vi "总磷总氮测量数据储存.vi"   [LabVIEW 2016, in "斯坦道通用流路CODmn.lvlib"]
uses:
  <vilib>/ptbypt/NI_PtbyPt.lvlib
types:
  T1 = cluster{"跨度值":dbl, "零点标准液浓度":dbl, "跨度标准液浓度":dbl, "标准液标准浓度":dbl}
  T2 = cluster{"系统时间":timestamp, "工作状态":u16, "测量模式":enum16{"待机", "连续模式", "周期模式", "定点模式", "受控模式", "手动模式"}, "告警代码":u16, "故障代码":u16, "日志代码":u16, "软件版本":u16, "F0":sgl, "F1":sgl, "F2":sgl, "F3":sgl, "T":sgl, "H":sgl, "id":u16, "flowid":u16, "量程":u16, "总磷控温温度1":sgl, "营养盐控温温度2":sgl, "ADC":sgl}
  T3 = cluster{"运行模式":enum16{"维护模式", "常规模式", "应急模式", "质控模式"}, "质控频次":enum16{"关闭", "每天", "星期一", "星期二", "星期三", "星期四", "星期五", "星期六", "星期日"}, "空白核查时间":u16, "跨度核查时间":u16, "测量间隔":u16}
  T4 = cluster{"总磷跨度值":dbl, "总磷零点标准液浓度":dbl, "总磷跨度标准液浓度":dbl, "总磷标准液标准浓度":dbl, "总氮跨度值":dbl, "总氮零点标准液浓度":dbl, "总氮跨度标准液浓度":dbl, "总氮标准液标准浓度":dbl, "COD跨度值":dbl, "COD零点标准液浓度":dbl, "COD跨度标准液浓度":dbl, "COD标准液标准浓度":dbl, "氨氮跨度值":dbl, "氨氮零点标准液浓度":dbl, "氨氮跨度标准液浓度":dbl, "氨氮标准液标准浓度":dbl, "磷酸盐跨度值":dbl, "磷酸盐零点标准液浓度":dbl, "磷酸盐跨度标准液浓度":dbl, "磷酸盐标准液标准浓度":dbl, "硝氮跨度值":dbl, "硝氮零点标准液浓度":dbl, "硝氮跨度标准液浓度":dbl, "硝氮标准液标准浓度":dbl, "亚硝氮跨度值":dbl, "亚硝氮零点标准液浓度":dbl, "亚硝氮跨度标准液浓度":dbl, "亚硝氮标准液标准浓度":dbl, "硫化物跨度值":dbl, "硫化物零点标准液浓度":dbl, "硫化物跨度标准液浓度":dbl, "硫化物标准液标准浓度":dbl, "硅酸盐跨度值":dbl, "硅酸盐零点标准液浓度":dbl, "硅酸盐跨度标准液浓度":dbl, "硅酸盐标准液标准浓度":dbl, "总磷零点标准液偏差":dbl, "总磷跨度标准液偏差":dbl, "总磷标准液标准偏差":dbl, "总氮零点标准液偏差":dbl, "总氮跨度标准液偏差":dbl, "总氮标准液标准偏差":dbl, "COD零点标准液偏差":dbl, "COD跨度标准液偏差":dbl, "COD标准液标准偏差":dbl, "氨氮零点标准液偏差":dbl, "氨氮跨度标准液偏差":dbl, "氨氮标准液标准偏差":dbl, "磷酸盐零点标准液偏差":dbl, "磷酸盐跨度标准液偏差":dbl, "磷酸盐标准液标准偏差":dbl, "硝氮零点标准液偏差":dbl, "硝氮跨度标准液偏差":dbl, "硝氮标准液标准偏差":dbl, "亚硝氮零点标准液偏差":dbl, "亚硝氮跨度标准液偏差":dbl, "亚硝氮标准液标准偏差":dbl, "硫化物零点标准液偏差":dbl, "硫化物跨度标准液偏差":dbl, "硫化物标准液标准偏差":dbl, "硅酸盐零点标准液偏差":dbl, "硅酸盐跨度标准液偏差":dbl, "硅酸盐标准液标准偏差":dbl, "氟化物跨度值":dbl, "氟化物零点标准液浓度":dbl, "氟化物跨度标准液浓度":dbl, "氟化物标准液标准浓度":dbl, "氟化物零点标准液偏差":dbl, "氟化物跨度标准液偏差":dbl, "氟化物标准液标准偏差":dbl, "CODMn跨度值":dbl, "CODMn零点标准液浓度":dbl, "CODMn跨度标准液浓度":dbl, "CODMn标准液标准浓度":dbl, "CODMn零点标准液偏差":dbl, "CODMn跨度标准液偏差":dbl, "CODMn标准液标准偏差":dbl}
  T5 = cluster{"因子编码":u32, "单位":u16, "标样参考值":sgl, "水样数据时间":timestamp, "水样实测值":sgl, "水样数据标识":string, "标样数据时间":timestamp, "标样实测值":sgl, "标样数据标识":string, "空白数据时间":timestamp, "空白实测值":sgl, "空白数据标识":string, "零点核查数据时间":timestamp, "零点核查实测值":sgl, "零点核查数据标识":string, "跨度核查数据时间":timestamp, "跨度核查实测值":sgl, "跨度核查数据标识":string, "加标回收数据时间":timestamp, "加标回收实测值":sgl, "加标回收数据标识":string, "平行样数据时间":timestamp, "平行样实测值":sgl, "平行样数据标识":string, "F0":sgl, "F1":sgl, "F2":sgl, "F3":sgl, "F4":sgl, "F5":sgl, "F6":sgl, "F7":sgl, "温度":sgl, "湿度":sgl, "X值":sgl, "fidrange":u16, "X1值":sgl}[]
  T6 = enum16{"水样测试", "标样核查", "跨度核查", "零点核查", "加标回收", "空白测试", "平行样"}[]
  T7 = cluster{"因子编码":u32, "单位":u16, "标样参考值":sgl, "水样数据时间":timestamp, "水样实测值":sgl, "水样数据标识":string, "标样数据时间":timestamp, "标样实测值":sgl, "标样数据标识":string, "空白数据时间":timestamp, "空白实测值":sgl, "空白数据标识":string, "零点核查数据时间":timestamp, "零点核查实测值":sgl, "零点核查数据标识":string, "跨度核查数据时间":timestamp, "跨度核查实测值":sgl, "跨度核查数据标识":string, "加标回收数据时间":timestamp, "加标回收实测值":sgl, "加标回收数据标识":string, "平行样数据时间":timestamp, "平行样实测值":sgl, "平行样数据标识":string, "F0":sgl, "F1":sgl, "F2":sgl, "F3":sgl, "F4":sgl, "F5":sgl, "F6":sgl, "F7":sgl, "温度":sgl, "湿度":sgl, "X值":sgl, "fidrange":u16, "X1值":sgl}
  T8 = cluster{"时间标识":timestamp, "测量模式":enum16{"维护数据", "水样测试", "标样核查", "零点核查", "跨度核查", "空白测试", "平行样测试", "加标回收", "空白校准", "标样校准", "初始化（清洗）", "快捷测试"}, "数据标记表":string, "监测值":sgl, "单位":u16, "数据标识":string, "因子编码":u32, "标样参考值":sgl, "F0":sgl, "F1":sgl, "F2":sgl, "F3":sgl, "F4":sgl, "F5":sgl, "F6":sgl, "F7":sgl, "X":sgl, "温度":sgl, "湿度":sgl, "量程标识":string, "SN":string, "跨度值":sgl, "X1":sgl}
  T9 = typedef "斯坦道通用流路CODmn.lvlib/关键参数.ctl" = cluster{"测量量程":sgl, "测量检出限":sgl, "测量精度":sgl, "测量间隔":sgl, "消解温度":sgl, "消解时长":sgl, "三项式系数":sgl, "二次多项式系数":sgl, "曲线斜率":sgl, "曲线截距":sgl, "线性相关系数":sgl, "空白校准时间":timestamp, "标样校准时间":timestamp, "测量信号值":sgl, "稀释倍数":sgl, "空白标定系数":sgl, "量程系数":sgl}
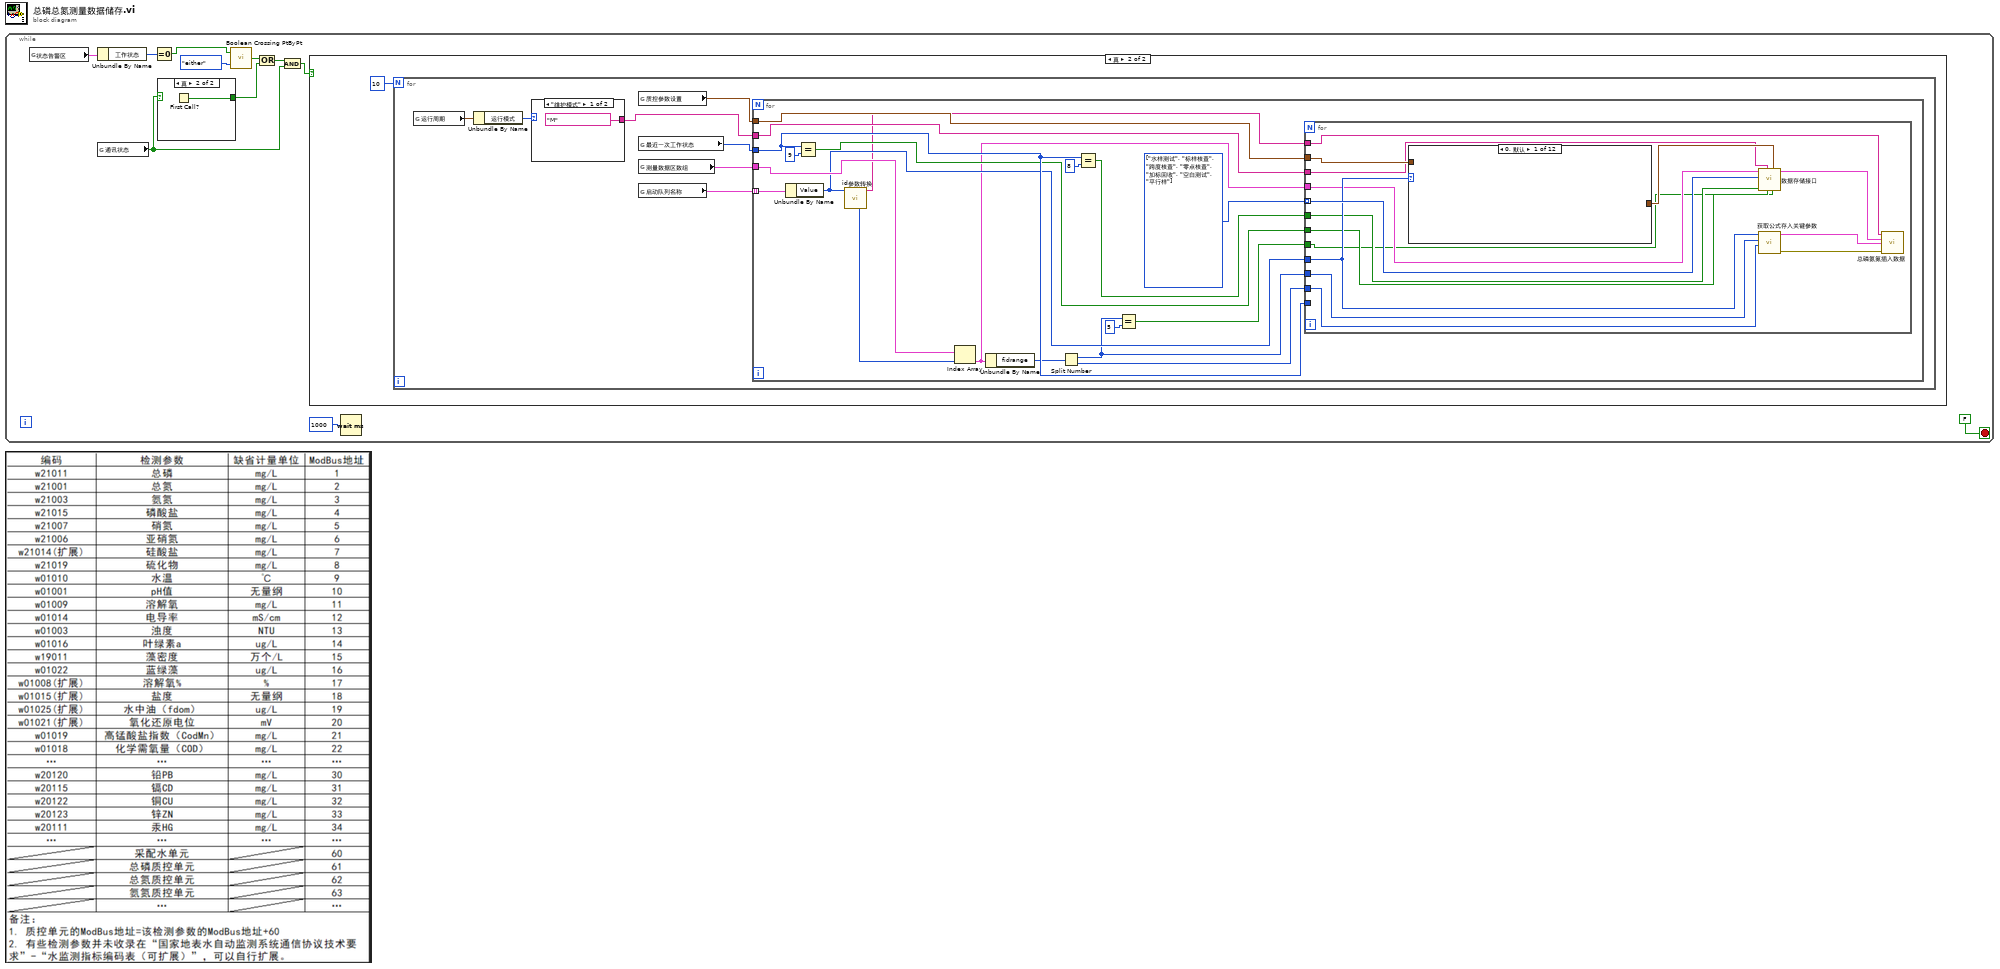
[diagram p0: block diagram]
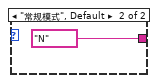
[diagram p4: hidden frame]
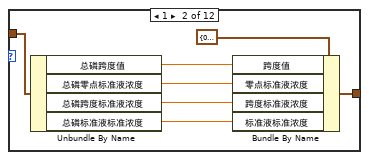
[diagram p5: hidden frame]
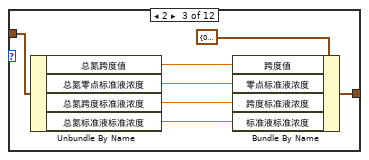
[diagram p6: hidden frame]
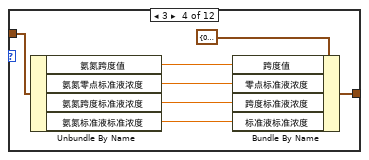
[diagram p7: hidden frame]
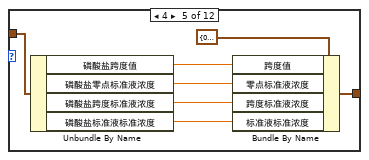
[diagram p8: hidden frame]
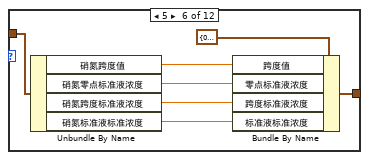
[diagram p9: hidden frame]
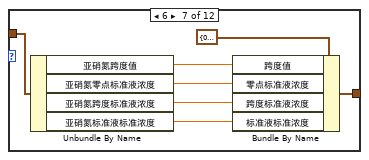
[diagram p10: hidden frame]
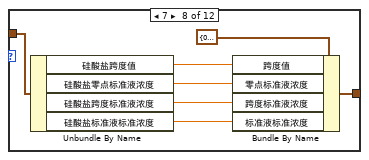
[diagram p11: hidden frame]
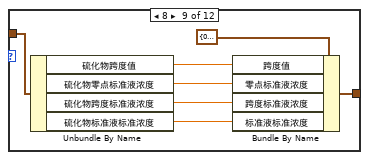
[diagram p12: hidden frame]
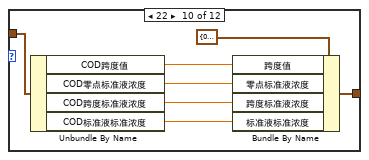
[diagram p13: hidden frame]
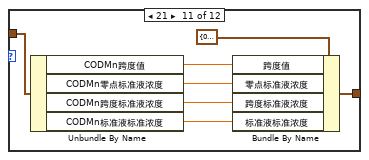
[diagram p14: hidden frame]
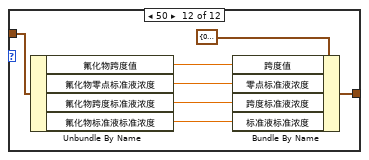
[diagram p15: hidden frame]
diagram:
  n1 = while {
    stop <- FALSE stop-if-true
    n2 = global read "VAR总磷总氮全局变量.vi" "状态告警区"() -> (w10:T2)
    n3 = Unbundle By Name(w10) -> ("工作状态"=w8:u16)
    n4 = global read "VAR总磷总氮全局变量.vi" "通讯状态"() -> (w3:bool)
    n5 = Equal To 0?(x=w8) -> (x = 0?=w5:bool)
    n6 = case shown="真" w3 {
      tunnel: [_ w12] -> w1
      frame False {
      }
      frame True {
        n7 = First Call?() -> (First Call?: T/F=w12:bool)
      }
    }
    n8 = call <vilib>:"Boolean Crossing PtByPt.vi"("direction"=enum16{"either", "false-true", "true-false"}."either", "input"=w5) -> ("crossing"=w6:bool)  [unwired: 1 in]
    n9 = Or(x=w6, y=w1) -> (x .or. y?=w2:bool)
    n10 = And(x=w2, y=w3) -> (x .and. y?=w4:bool)
    n11 = case shown="真" w4 {
      frame False {
      }
      frame True {
        n12 = for {
          N: 10 -> [_]
          n13 = global read "总磷总氮断电保存全局变量.vi" "运行周期"() -> (w16:T3)
          n14 = Unbundle By Name(w16) -> ("运行模式"=w15:enum16{"维护模式", "常规模式", "应急模式", "质控模式"})
          n15 = case shown="\"维护模式\"" w15 {
            tunnel: ["M" ("数据标记表") "N" ("数据标记表")] -> w14
            frame "维护模式" {
            }
            frame "常规模式", Default {
            }
          }
          n16 = global read "总磷总氮断电保存全局变量.vi" "质控参数设置"() -> (w17:T4)
          n17 = global read "VAR总磷总氮全局变量.vi" "最近一次工作状态"() -> (w19:u16)
          n18 = global read "VAR总磷总氮全局变量.vi" "测量数据区数组"() -> (w18:T5)
          n19 = global read "model config var.vi" "启动队列名称"() -> (w20:cluster{"String":string, "Value":u16}[])
          n20 = for {
            tunnel: w20 -> [w38] mode=indexing
            tunnel: w19 -> [w34]
            tunnel: w18 -> [w32]
            tunnel: w17 -> [w40]
            tunnel: w14 -> [w39]
            w41 = T6 [enum."水样测试", enum."标样核查", enum."跨度核查", enum."零点核查", enum."加标回收", enum."空白测试", enum."平行样"] items=["水样测试", "标样核查", "跨度核查", "零点核查", "加标回收", "空白测试", "平行样"]
            n21 = Unbundle By Name(w38) -> ("Value"=w31:u16)
            n22 = Equal?(x=w34, y=u16 9) -> (x = y?=w33:bool)
            n23 = call "id参数转换.vi"("id"=w31) -> ("table输出"=w30:string, "数组资源索引"=w23:i32)  [unwired: 9 in]
            n24 = Index Array(array=w32, index=w23) -> (element=w27:T7)
            n25 = Unbundle By Name(w27) -> ("fidrange"=w29:u16)
            n26 = Split Number(x=w29) -> (hi(x)=w24:u8, lo(x)=w25:u8)
            n27 = Equal?(x=w34, y=u16 8) -> (x = y?=w36:bool)
            n28 = Equal?(x=w24, y=u16 5) -> (x = y?=w26:bool)
            n29 = for {
              tunnel: w41 -> [w53] mode=indexing
              tunnel: w34 -> [_]
              tunnel: w40 -> [w51]
              tunnel: w39 -> [w50]
              tunnel: w31 -> [w49]
              tunnel: w36 -> [w48]
              tunnel: w33 -> [w47]
              tunnel: w27 -> [w46]
              tunnel: w30 -> [w45]
              tunnel: w26 -> [w44]
              tunnel: w25 -> [w43]
              tunnel: w24 -> [w42]
              n30 = case shown="0, 默认" w49 {
                tunnel: w51 -> [_ w63 w70 w77 w84 w91 w98 w105 w112 w119 w126 w133]
                tunnel: [_ w61 w68 w75 w82 w89 w96 w103 w110 w117 w124 w131] -> w55
                frame 0, Default {
                }
                frame 1 {
                  n31 = Unbundle By Name(w63) -> ("总磷跨度值"=w60:dbl, "总磷零点标准液浓度"=w59:dbl, "总磷跨度标准液浓度"=w58:dbl, "总磷标准液标准浓度"=w57:dbl)
                  n32 = Bundle By Name(cluster=T1 {"跨度值"=0.0, "零点标准液浓度"=0.0, "跨度标准液浓度"=0.0, "标准液标准浓度"=0.0} ("质控参数设置"), "跨度值"=w60, "零点标准液浓度"=w59, "跨度标准液浓度"=w58, "标准液标准浓度"=w57) -> (w61:T1)
                }
                frame 2 {
                  n33 = Unbundle By Name(w70) -> ("总氮跨度值"=w67:dbl, "总氮零点标准液浓度"=w66:dbl, "总氮跨度标准液浓度"=w65:dbl, "总氮标准液标准浓度"=w64:dbl)
                  n34 = Bundle By Name(cluster=T1 {"跨度值"=0.0, "零点标准液浓度"=0.0, "跨度标准液浓度"=0.0, "标准液标准浓度"=0.0} ("质控参数设置"), "跨度值"=w67, "零点标准液浓度"=w66, "跨度标准液浓度"=w65, "标准液标准浓度"=w64) -> (w68:T1)
                }
                frame 3 {
                  n35 = Unbundle By Name(w77) -> ("氨氮跨度值"=w74:dbl, "氨氮零点标准液浓度"=w73:dbl, "氨氮跨度标准液浓度"=w72:dbl, "氨氮标准液标准浓度"=w71:dbl)
                  n36 = Bundle By Name(cluster=T1 {"跨度值"=0.0, "零点标准液浓度"=0.0, "跨度标准液浓度"=0.0, "标准液标准浓度"=0.0} ("质控参数设置"), "跨度值"=w74, "零点标准液浓度"=w73, "跨度标准液浓度"=w72, "标准液标准浓度"=w71) -> (w75:T1)
                }
                frame 4 {
                  n37 = Unbundle By Name(w84) -> ("磷酸盐跨度值"=w81:dbl, "磷酸盐零点标准液浓度"=w80:dbl, "磷酸盐跨度标准液浓度"=w79:dbl, "磷酸盐标准液标准浓度"=w78:dbl)
                  n38 = Bundle By Name(cluster=T1 {"跨度值"=0.0, "零点标准液浓度"=0.0, "跨度标准液浓度"=0.0, "标准液标准浓度"=0.0} ("质控参数设置"), "跨度值"=w81, "零点标准液浓度"=w80, "跨度标准液浓度"=w79, "标准液标准浓度"=w78) -> (w82:T1)
                }
                frame 5 {
                  n39 = Unbundle By Name(w91) -> ("硝氮跨度值"=w88:dbl, "硝氮零点标准液浓度"=w87:dbl, "硝氮跨度标准液浓度"=w86:dbl, "硝氮标准液标准浓度"=w85:dbl)
                  n40 = Bundle By Name(cluster=T1 {"跨度值"=0.0, "零点标准液浓度"=0.0, "跨度标准液浓度"=0.0, "标准液标准浓度"=0.0} ("质控参数设置"), "跨度值"=w88, "零点标准液浓度"=w87, "跨度标准液浓度"=w86, "标准液标准浓度"=w85) -> (w89:T1)
                }
                frame 6 {
                  n41 = Unbundle By Name(w98) -> ("亚硝氮跨度值"=w95:dbl, "亚硝氮零点标准液浓度"=w94:dbl, "亚硝氮跨度标准液浓度"=w93:dbl, "亚硝氮标准液标准浓度"=w92:dbl)
                  n42 = Bundle By Name(cluster=T1 {"跨度值"=0.0, "零点标准液浓度"=0.0, "跨度标准液浓度"=0.0, "标准液标准浓度"=0.0} ("质控参数设置"), "跨度值"=w95, "零点标准液浓度"=w94, "跨度标准液浓度"=w93, "标准液标准浓度"=w92) -> (w96:T1)
                }
                frame 7 {
                  n43 = Unbundle By Name(w105) -> ("硅酸盐跨度值"=w102:dbl, "硅酸盐零点标准液浓度"=w101:dbl, "硅酸盐跨度标准液浓度"=w100:dbl, "硅酸盐标准液标准浓度"=w99:dbl)
                  n44 = Bundle By Name(cluster=T1 {"跨度值"=0.0, "零点标准液浓度"=0.0, "跨度标准液浓度"=0.0, "标准液标准浓度"=0.0} ("质控参数设置"), "跨度值"=w102, "零点标准液浓度"=w101, "跨度标准液浓度"=w100, "标准液标准浓度"=w99) -> (w103:T1)
                }
                frame 8 {
                  n45 = Unbundle By Name(w112) -> ("硫化物跨度值"=w109:dbl, "硫化物零点标准液浓度"=w108:dbl, "硫化物跨度标准液浓度"=w107:dbl, "硫化物标准液标准浓度"=w106:dbl)
                  n46 = Bundle By Name(cluster=T1 {"跨度值"=0.0, "零点标准液浓度"=0.0, "跨度标准液浓度"=0.0, "标准液标准浓度"=0.0} ("质控参数设置"), "跨度值"=w109, "零点标准液浓度"=w108, "跨度标准液浓度"=w107, "标准液标准浓度"=w106) -> (w110:T1)
                }
                frame 22 {
                  n47 = Unbundle By Name(w119) -> ("COD跨度值"=w116:dbl, "COD零点标准液浓度"=w115:dbl, "COD跨度标准液浓度"=w114:dbl, "COD标准液标准浓度"=w113:dbl)
                  n48 = Bundle By Name(cluster=T1 {"跨度值"=0.0, "零点标准液浓度"=0.0, "跨度标准液浓度"=0.0, "标准液标准浓度"=0.0} ("质控参数设置"), "跨度值"=w116, "零点标准液浓度"=w115, "跨度标准液浓度"=w114, "标准液标准浓度"=w113) -> (w117:T1)
                }
                frame 21 {
                  n49 = Unbundle By Name(w126) -> ("CODMn跨度值"=w123:dbl, "CODMn零点标准液浓度"=w122:dbl, "CODMn跨度标准液浓度"=w121:dbl, "CODMn标准液标准浓度"=w120:dbl)
                  n50 = Bundle By Name(cluster=T1 {"跨度值"=0.0, "零点标准液浓度"=0.0, "跨度标准液浓度"=0.0, "标准液标准浓度"=0.0} ("质控参数设置"), "跨度值"=w123, "零点标准液浓度"=w122, "跨度标准液浓度"=w121, "标准液标准浓度"=w120) -> (w124:T1)
                }
                frame 50 {
                  n51 = Unbundle By Name(w133) -> ("氟化物跨度值"=w130:dbl, "氟化物零点标准液浓度"=w129:dbl, "氟化物跨度标准液浓度"=w128:dbl, "氟化物标准液标准浓度"=w127:dbl)
                  n52 = Bundle By Name(cluster=T1 {"跨度值"=0.0, "零点标准液浓度"=0.0, "跨度标准液浓度"=0.0, "标准液标准浓度"=0.0} ("质控参数设置"), "跨度值"=w130, "零点标准液浓度"=w129, "跨度标准液浓度"=w128, "标准液标准浓度"=w127) -> (w131:T1)
                }
              }
              n53 = call "数据存储接口.vi"("快捷测试？"=w44, "质控参数设置"=w55, "标样校准？"=w47, "数据标记表"=w50, "空白校准？"=w48, "数据存储模式"=w53, "测量数据区"=w46) -> ("data输出"=w56:T8)  [unwired: 4 in]
              n54 = call "获取公式存入关键参数.vi"("量程"=w43, "flowid"=w42, "id"=w49) -> ("error out"=w54:errorcluster, "关键参数"=w52:T9)  [unwired: 7 in]
              n55 = call "总磷氨氮插入数据.vi"("table"=w45, "data"=w56, "关键参数"=w52, "error in (no error)"=w54) -> ()  [unwired: 11 in, 1 out]
            }
          }
        }
      }
    }
    n56 = Wait (ms)(milliseconds to wait=u32 1000 ("等待时间（毫秒）")) -> ()  [unwired: 1 out]
  }
